vi "Begin.vi"() -> (1 "CameraDevRef":T5)   [LabVIEW 2011]
doc: "Called before other user functions, this VI is expected to open initial I/O refnums, load in file data, and do all program initialization. Notice that the <B>error out</B> terminal is simply used for data flow. Wiring it to other structures or subVIs ensures that this VI runs first."
uses:
  <vilib>/Rock Robotics/WPI/Camera/WPI_CameraDevRef.ctl
  <vilib>/Rock Robotics/WPI/Encoder/WPI_EncoderDevRef.ctl
  <vilib>/Rock Robotics/SystemInterfaces/Encoder/FPGA_EncoderIdx.ctl
  <vilib>/Rock Robotics/SystemInterfaces/Counter/FPGA_CounterCtrSystemIndex.ctl
  <vilib>/Rock Robotics/WPI/Encoder/WPI_EncoderType.ctl
  <vilib>/Rock Robotics/WPI/Joystick/WPI_JoystickDeviceEnum.ctl
  <vilib>/Rock Robotics/SystemInterfaces/DIO/FPGA_DIOPWMChannel.ctl
  <vilib>/Rock Robotics/SystemInterfaces/Typedef/FPGA_TypedefDigitalModule.ctl
  <vilib>/Rock Robotics/WPI/MotorControl/WPI_MotorControlOpen Victor.vi
  Robot Global Data.vi
  <vilib>/Rock Robotics/SystemInterfaces/DIO/FPGA_DIORelayChannel.ctl
  <vilib>/Rock Robotics/WPI/Relay/WPI_RelayDirection.ctl
  <vilib>/Rock Robotics/SystemInterfaces/AI/FPGA_AIChannel.ctl
  <vilib>/Rock Robotics/WPI/Counter/WPI_CounterDigitalInputToDigitalSource.vi
  <vilib>/Rock Robotics/SystemInterfaces/DIO/FPGA_DIOChannel.ctl
  <vilib>/Rock Robotics/SystemInterfaces/AI/FPGA_AIGyroChannel.ctl
  <vilib>/Rock Robotics/WPI/MotorControl/WPI_MotorControlOpen Jaguar.vi
  <vilib>/Rock Robotics/SystemInterfaces/Typedef/FPGA_TypedefAnalogModule.ctl
  <vilib>/Utility/file.llb/Read From Spreadsheet File (DBL).vi
panel:
  out "LDriveEncoder 3":cluster{"status":bool}
  out "EncoderDevRef 3":T1={"DevStatus"={"status"=FALSE, "code"=0, "source"=""}, "EncoderIndex"=enum."Invalid", "CounterIndex"=enum."Invalid", "DistancePerCount"=1.0, "Decoding Type"=enum."4x"}
  out "EncoderDevRef 2":T1={"DevStatus"={"status"=FALSE, "code"=0, "source"=""}, "EncoderIndex"=enum."Invalid", "CounterIndex"=enum."Invalid", "DistancePerCount"=1.0, "Decoding Type"=enum."4x"}
  out "LDriveEncoder 2":errorcluster
  out "EncoderDevRef":T1={"DevStatus"={"status"=FALSE, "code"=0, "source"=""}, "EncoderIndex"=enum."Invalid", "CounterIndex"=enum."Invalid", "DistancePerCount"=1.0, "Decoding Type"=enum."4x"}
  out "LDriveEncoder":errorcluster
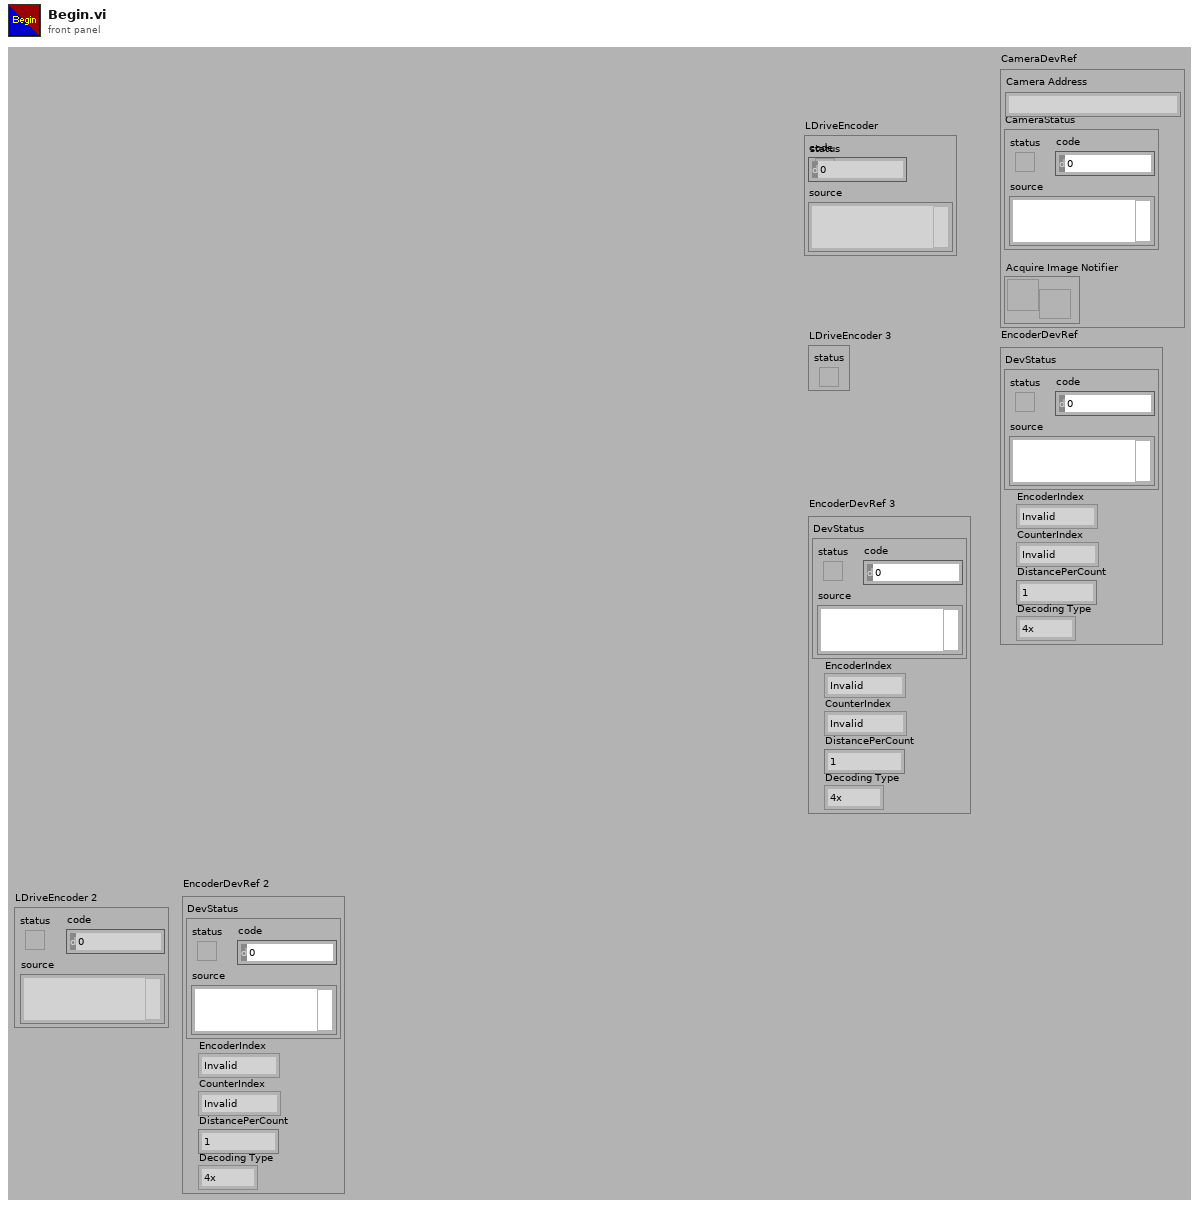
[diagram p1: front panel]
types:
  T1 = typedef "WPI_EncoderDevRef.ctl" = cluster{"DevStatus":errorcluster, "EncoderIndex":T2, "CounterIndex":T3, "DistancePerCount":dbl, "Decoding Type":T4}
  T2 = typedef "FPGA_EncoderIdx.ctl" = enum8{"Enc 0", "Enc 1", "Enc 2", "Enc 3", "Invalid"}
  T3 = typedef "FPGA_CounterCtrSystemIndex.ctl" = enum8{"Ctr 0", "Ctr 1", "Ctr 2", "Ctr 3", "Ctr 4", "Ctr 5", "Ctr 6", "Ctr 7", "Invalid"}
  T4 = typedef "WPI_EncoderType.ctl" = enum16{"1x", "2x", "4x"}
  T5 = typedef "WPI_CameraDevRef.ctl" = cluster{"Camera Address":string, "CameraStatus":errorcluster, "Acquire Image Notifier":refnum<notifier>}
  T6 = typedef "FPGA_TypedefDigitalModule.ctl" = enum16{"Digital Module 1", "Digital Module 2"}
  T7 = typedef "FPGA_DIOPWMChannel.ctl" = enum8{"PWM 1", "PWM 2", "PWM 3", "PWM 4", "PWM 5", "PWM 6", "PWM 7", "PWM 8", "PWM 9", "PWM 10", "Invalid"}
  T8 = typedef "WPI_JoystickDeviceEnum.ctl" = enum16{"USB 1", "USB 2", "USB 3", "USB 4", "Kinect 1", "Kinect 2"}
  T9 = typedef "FPGA_DIORelayChannel.ctl" = enum8{"Relay 1", "Relay 2", "Relay 3", "Relay 4", "Relay 5", "Relay 6", "Relay 7", "Relay 8", "Invalid"}
  T10 = typedef "FPGA_DIOChannel.ctl" = enum8{"DIO 1", "DIO 2", "DIO 3", "DIO 4", "DIO 5", "DIO 6", "DIO 7", "DIO 8", "DIO 9", "DIO 10", "DIO 11", "DIO 12", "DIO 13", "DIO 14", "Invalid"}
  T11 = typedef "WPI_MotorControlDeviceRef.ctl" = cluster{"DeviceStatus":errorcluster, "Type":enum16{"PWM", "CAN"}, "PWM":cluster{"Digital Module":T6, "PWM Channel":T7, "DeadBand":T12}, "CAN":cluster{"Device Number":u8, "Control Mode":T13, "Semaphore":T14, "Max Vout":dbl}, "Invert":bool, "TransformRef":T15, "InvTransformRef":T15}
  T12 = typedef "WPI_PWMDeadband.ctl" = cluster{"Name":string, "maxPositivePwm":i32, "minPositivePwm":i32, "centerPwm":i32, "maxNegativePwm":i32, "minNegativePwm":i32, "angularRange":u16}
  T13 = typedef "WPI_CANJaguar_ControlMode.ctl" = enum8{"Percent VBus", "Current", "Speed", "Position", "Voltage"}
  T14 = typedef "Semaphore RefNum" = refnum<k1>
  T15 = typedef "WPI_PWMTransform_ConPane.ctl" = refnum<vi>
  T16 = typedef "WPI_DigitalInputDevRef.ctl" = cluster{"DevStatus":errorcluster, "DIO Channel":T10, "Digital Module":T6}
  T17 = typedef "FPGA_CounterEncoderSourceConvertionLVSourceType.ctl" = cluster{"DevStatus":errorcluster, "AnalogTriggerMode?":bool, "DigitalMode":cluster{"Digital Module":T6, "DIO Channel":T18}, "AnalogTriggerMode":cluster{"AnalogTriggerIndex":T19, "OutputType":T20}}
  T18 = typedef "FPGA_DIODigitalSourceChannel.ctl" = enum8{"DIO 1", "DIO 2", "DIO 3", "DIO 4", "DIO 5", "DIO 6", "DIO 7", "DIO 8", "DIO 9", "DIO 10", "DIO 11", "DIO 12", "DIO 13", "DIO 14", "Disabled"}
  T19 = typedef "FPGA_AnalogTriggerIndex.ctl" = enum8{"Trig 0", "Trig 1", "Trig 2", "Trig 3", "Trig 4", "Trig 5", "Trig 6", "Trig 7", "Invalid"}
  T20 = typedef "FPGA_AnalogTriggerOutType.ctl" = enum16{"InWindow", "TriggerState", "Rising", "Falling"}
  T21 = typedef "WPI_RelayDevRef.ctl" = cluster{"DevStatus":errorcluster, "Relay Channel":T9, "Digital Module":T6, "Relay Direction":T22}
  T22 = typedef "WPI_RelayDirection.ctl" = enum16{"Both directions", "Forward only", "Reverse only"}
  T23 = typedef "FPGA_AIChannel.ctl" = enum8{"AI 1", "AI 2", "AI 3", "AI 4", "AI 5", "AI 6", "AI 7", "AI 8", "Invalid"}
  T24 = typedef "WPI_AnalogChannelDevRef.ctl" = cluster{"DevStatus":errorcluster, "Analog Module":T25, "Analog Channel":T23}
  T25 = typedef "FPGA_TypedefAnalogModule.ctl" = enum16{"Analog Module 1", "Analog Module 2"}
  T26 = typedef "WPI_CameraImageSize.ctl" = enum16{"640x480", "320x240", "160x120"}
  T27 = cluster{"fps":i32, "compression":i32, "Image Size":T26}
  T28 = typedef "WPI_CameraWhite Balance Values.ctl" = enum16{"Auto", "Fixed indoor", "Fixed outdoor 1", "Fixed outdoor 2", "Fixed fluorescent 1", "Fixed fluorescent 2", "Hold current"}
  T29 = typedef "WPI_CameraExposure Values.ctl" = enum16{"Auto", "Flicker-free 50 Hz", "Flicker-free 60 Hz", "Hold current"}
  T30 = typedef "WPI_ServoDeviceRef.ctl" = cluster{"DeviceStatus":errorcluster, "Digital Module":T6, "PWM Channel":T7, "DeadBand":T12}
  T31 = typedef "WPI_JoystickDevRef.ctl" = cluster{"Device":T8}
  T32 = typedef "FPGA_AIGyroChannel.ctl" = enum8{"AI 1", "AI 2", "Invalid"}
  T33 = typedef "WPI_GyroDevRef.ctl" = cluster{"DevStatus":errorcluster, "Analog Module":T25, "Analog Channel":T23, "Offset":dbl, "Gain (VoltsPerDegree/Second)":dbl}
  T34 = typedef "WPI_UltrasonicDeviceRef.ctl" = cluster{"DevStatus":errorcluster, "Ping Digital Module":T6, "Echo Digital Module":T6, "Ping Channel":T10, "Echo Channel":T10, "CntIndex":T3}
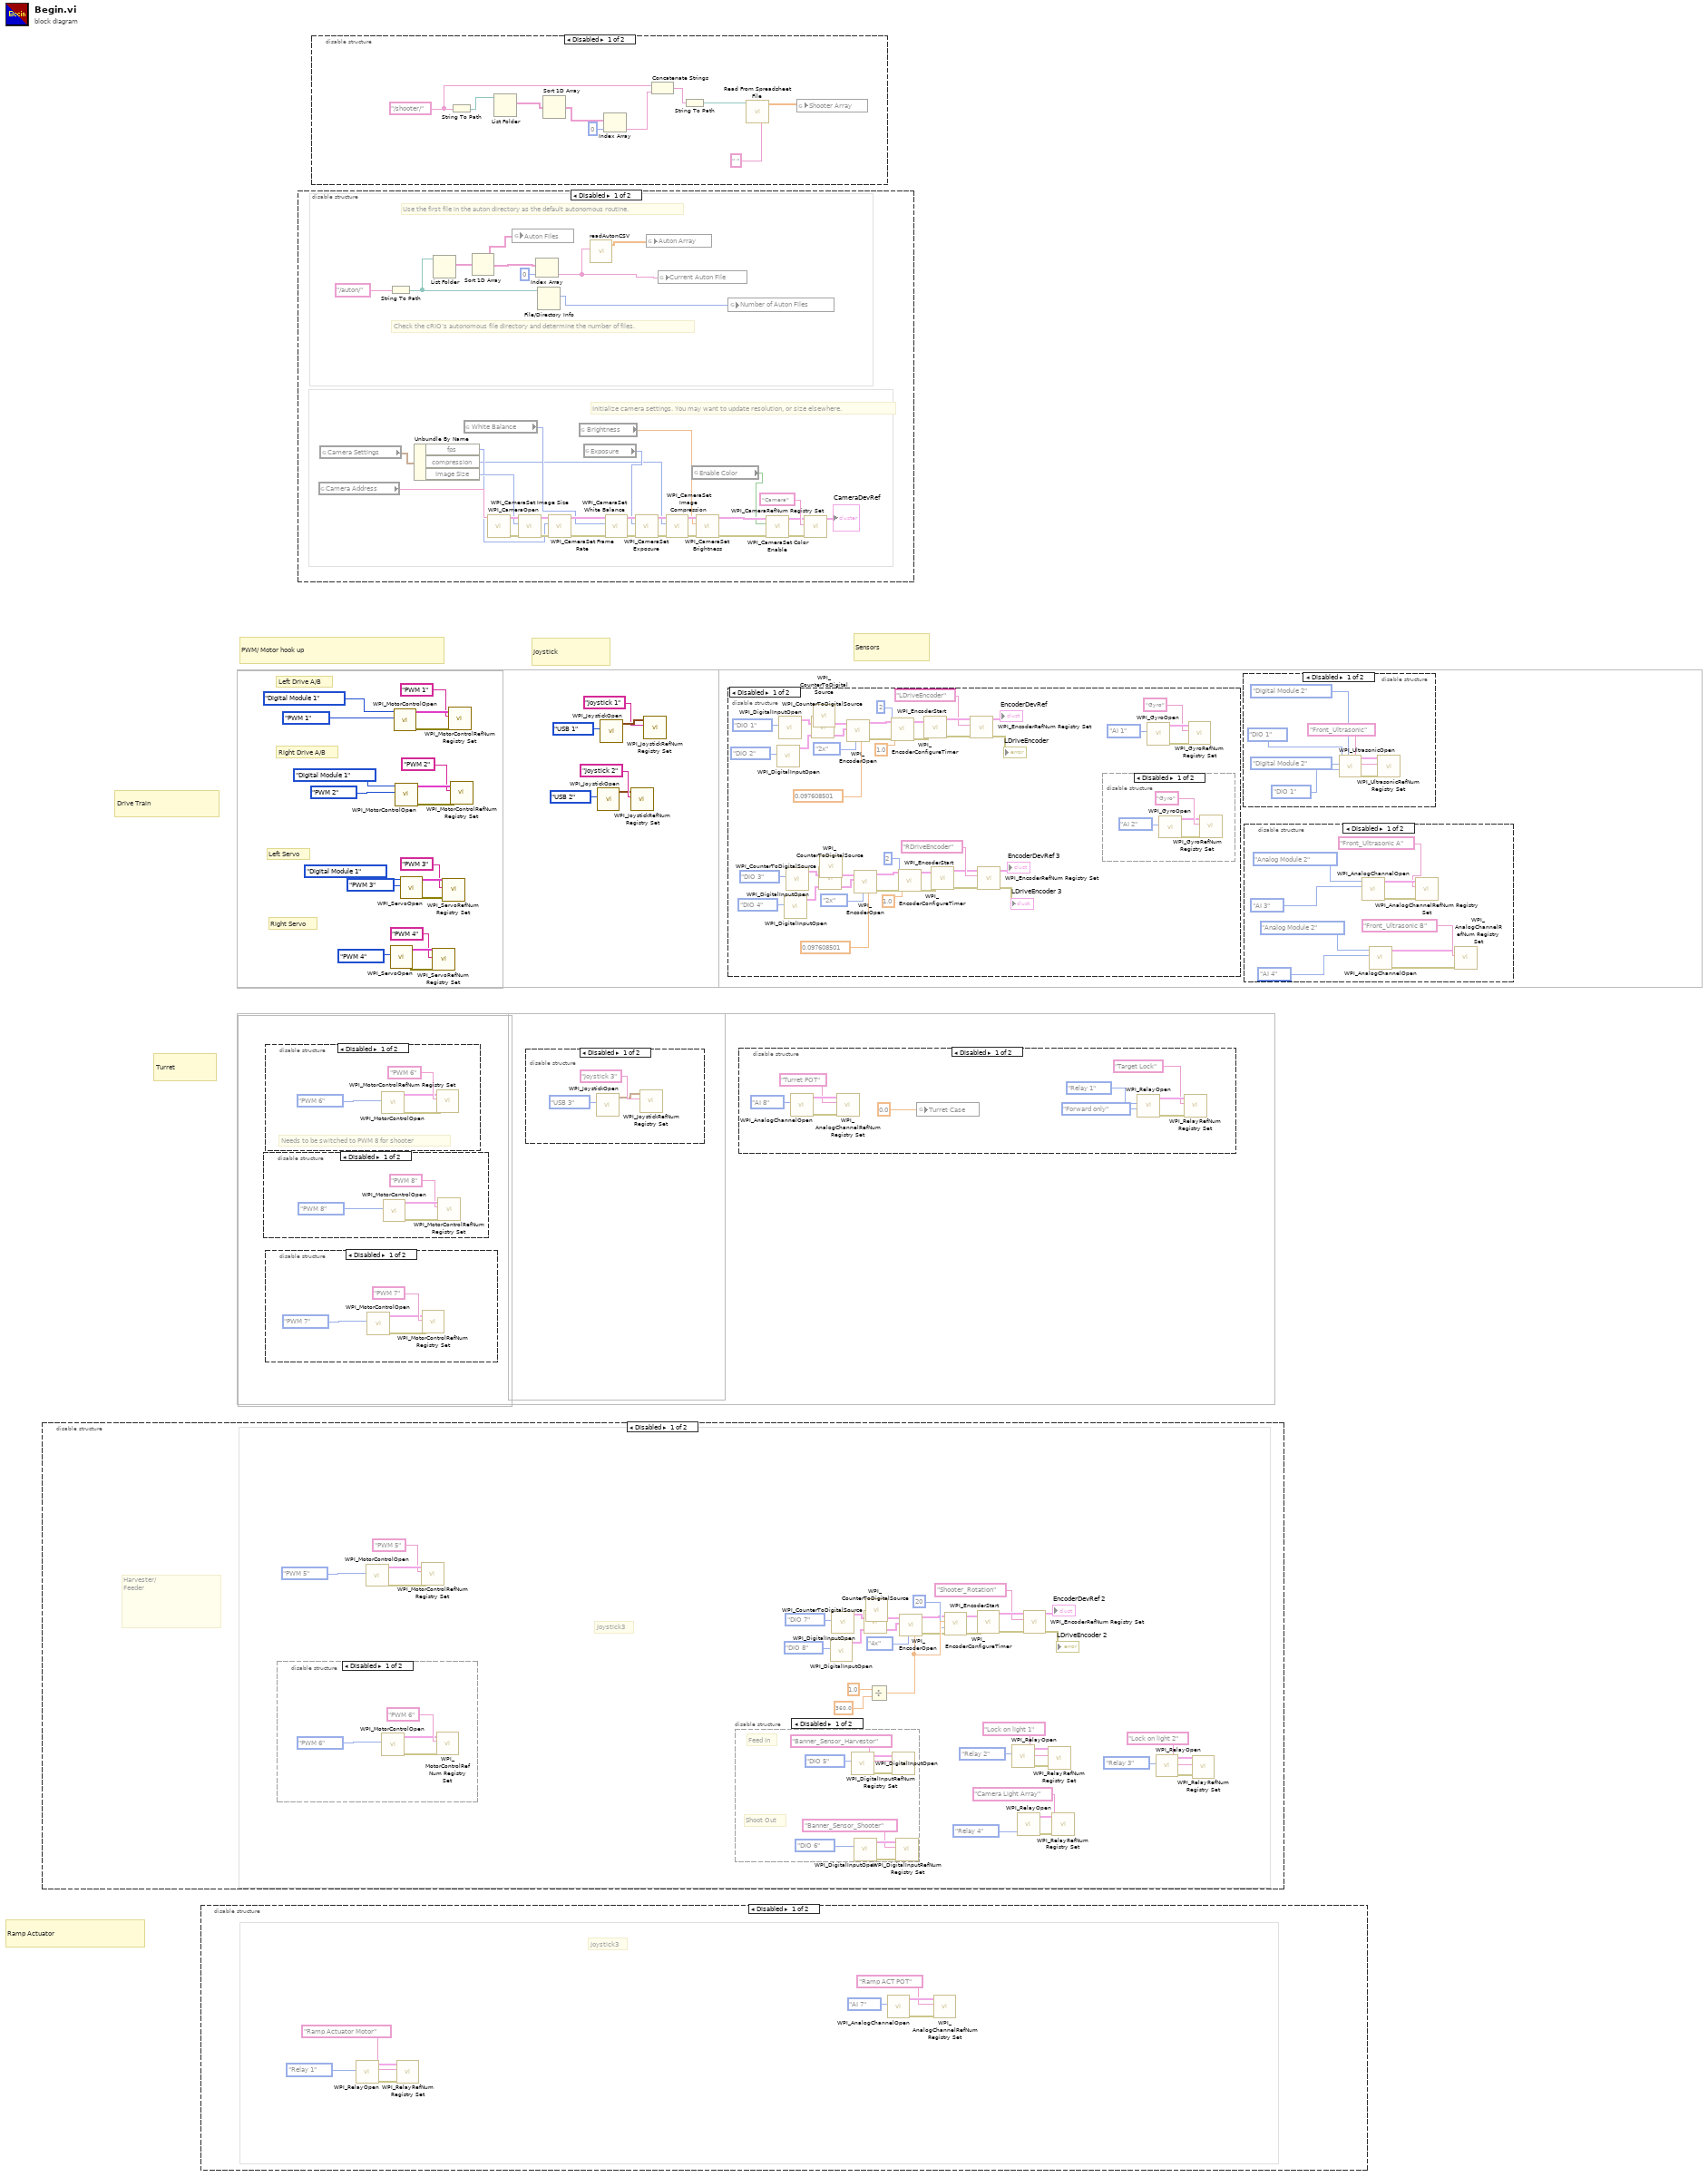
[diagram p0: block diagram]
diagram:
  # "Right Drive A/B"
  # "Left Drive A/B"
  # "Right Servo"
  # "Left Servo"
  # "Turret"
  # "Ramp Actuator"
  # "Drive Train"
  # "Sensors"
  # "Joystick"
  # "PWM/ Motor hook up"
  n1 = disable-structure shown="Disabled" {
    frame Disabled {
      # "Harvester/\nFeeder"
      # "Joystick3"
      n2 = disable-structure shown="Disabled" {
        frame Disabled {
          n3 = call-poly <vilib>:"WPI_MotorControlOpen.vi"("PWM Channel"=FPGA_DIOPWMChannel."PWM 6") -> ("error out"=w73:errorcluster, "MotorControlDeviceRef"=w71:T11)  [unwired: 9 in]
          n4 = call <vilib>:"WPI_MotorControlRefNum Registry Set.vi"("error in (no error)"=w73, "refnum name"="PWM 6", "MotorControlDevRef"=w71) -> ()  [unwired: 7 in, 2 out]
        }
        frame Enabled {
        }
      }
      n5 = call-poly <vilib>:"WPI_MotorControlOpen.vi"("PWM Channel"=FPGA_DIOPWMChannel."PWM 5") -> ("error out"=w58:errorcluster, "MotorControlDeviceRef"=w60:T11)  [unwired: 9 in]
      n6 = call <vilib>:"WPI_MotorControlRefNum Registry Set.vi"("error in (no error)"=w58, "refnum name"="PWM 5", "MotorControlDevRef"=w60) -> ()  [unwired: 7 in, 2 out]
      n7 = disable-structure shown="Disabled" {
        frame Disabled {
          # "Shoot Out"
          # "Feed in"
          n8 = call <vilib>:"WPI_DigitalInputOpen.vi"("DIO Channel"=FPGA_DIOChannel."DIO 5") -> ("error out"=w67:errorcluster, "DigitalInputDevRef"=w66:T16)  [unwired: 9 in]
          n9 = call <vilib>:"WPI_DigitalInputOpen.vi"("DIO Channel"=FPGA_DIOChannel."DIO 6") -> ("error out"=w64:errorcluster, "DigitalInputDevRef"=w63:T16)  [unwired: 9 in]
          n10 = call <vilib>:"WPI_DigitalInputRefNum Registry Set.vi"("error in (no error)"=w67, "refnum name"="Banner_Sensor_Harvestor", "DigitalInputDevRef"=w66) -> ()  [unwired: 7 in, 2 out]
          n11 = call <vilib>:"WPI_DigitalInputRefNum Registry Set.vi"("error in (no error)"=w64, "refnum name"="Banner_Sensor_Shooter", "DigitalInputDevRef"=w63) -> ()  [unwired: 7 in, 2 out]
        }
        frame Enabled {
        }
      }
      n12 = call <vilib>:"WPI_DigitalInputOpen.vi"("DIO Channel"=FPGA_DIOChannel."DIO 8") -> ("DigitalInputDevRef"=w42:T16)  [unwired: 9 in, 1 out]
      n13 = call <vilib>:"WPI_DigitalInputOpen.vi"("DIO Channel"=FPGA_DIOChannel."DIO 7") -> ("DigitalInputDevRef"=w39:T16)  [unwired: 9 in, 1 out]
      n14 = call-poly <vilib>:"WPI_CounterToDigitalSource.vi"("DigitalInputDevRef"=w42) -> ("Digital Source"=w43:T17)  [unwired: 6 in]
      n15 = call-poly <vilib>:"WPI_CounterToDigitalSource.vi"("DigitalInputDevRef"=w39) -> ("Digital Source"=w38:T17)  [unwired: 6 in]
      n16 = Divide(x=1.0, y=360.0) -> (x/y=w57:dbl)
      n17 = call <vilib>:"WPI_EncoderOpen.vi"("DistancePerCount"=w57, "Decoding Type"=WPI_EncoderType."4x", "BSource"=w43, "ASource"=w38) -> ("error out"=w46:errorcluster, "EncoderDevRef"=w47:T1)  [unwired: 6 in]
      n18 = call <vilib>:"WPI_EncoderConfigureTimer.vi"("error in (no error)"=w46, "Number Samples to Average"=u8 20, "Minimum Rate"=w57, "EncoderDevRef"=w47) -> ("error out"=w50:errorcluster, "EncoderDevRef"=w49:T1)  [unwired: 6 in]
      n19 = call <vilib>:"WPI_EncoderStart.vi"("error in (no error)"=w50, "EncoderDevRef"=w49) -> ("error out"=w52:errorcluster, "EncoderDevRef"=w51:T1)  [unwired: 8 in]
      n20 = call <vilib>:"WPI_RelayOpen.vi"("Relay Channel"=FPGA_DIORelayChannel."Relay 2") -> ("error out"=w35:errorcluster, "RelayDevRef"=w34:T21)  [unwired: 9 in]
      n21 = call <vilib>:"WPI_RelayOpen.vi"("Relay Channel"=FPGA_DIORelayChannel."Relay 4") -> ("error out"=w37:errorcluster, "RelayDevRef"=w36:T21)  [unwired: 9 in]
      n22 = call <vilib>:"WPI_EncoderRefNum Registry Set.vi"("error in (no error)"=w52, "refnum name"="Shooter_Rotation", "EncoderDevRef"=w51) -> ("error out"=→"LDriveEncoder 2":errorcluster, "EncoderDevRef"=→"EncoderDevRef 2":T1)  [unwired: 7 in]
      n23 = call <vilib>:"WPI_RelayRefNum Registry Set.vi"("error in (no error)"=w35, "refnum name"="Lock on light 1", "RelayDevRef"=w34) -> ()  [unwired: 7 in, 2 out]
      n24 = call <vilib>:"WPI_RelayRefNum Registry Set.vi"("error in (no error)"=w37, "refnum name"="Camera Light Array", "RelayDevRef"=w36) -> ()  [unwired: 7 in, 2 out]
      n25 = call <vilib>:"WPI_RelayOpen.vi"("Relay Channel"=FPGA_DIORelayChannel."Relay 3") -> ("error out"=w26:errorcluster, "RelayDevRef"=w27:T21)  [unwired: 9 in]
      n26 = call <vilib>:"WPI_RelayRefNum Registry Set.vi"("error in (no error)"=w26, "refnum name"="Lock on light 2", "RelayDevRef"=w27) -> ()  [unwired: 7 in, 2 out]
    }
    frame Enabled {
    }
  }
  n27 = disable-structure shown="Disabled" {
    frame Disabled {
      # "Joystick3"
      n28 = call <vilib>:"WPI_RelayOpen.vi"("Relay Channel"=FPGA_DIORelayChannel."Relay 1") -> ("error out"=w77:errorcluster, "RelayDevRef"=w76:T21)  [unwired: 9 in]
      n29 = call <vilib>:"WPI_RelayRefNum Registry Set.vi"("error in (no error)"=w77, "refnum name"="Ramp Actuator Motor", "RelayDevRef"=w76) -> ()  [unwired: 7 in, 2 out]
      n30 = call <vilib>:"WPI_AnalogChannelOpen.vi"("Analog Channel"=FPGA_AIChannel."AI 7") -> ("error out"=w80:errorcluster, "AIDeviceRef"=w81:T24)  [unwired: 9 in]
      n31 = call <vilib>:"WPI_AnalogChannelRefNum Registry Set.vi"("error in (no error)"=w80, "refnum name"="Ramp ACT POT", "AIDeviceRef"=w81) -> ()  [unwired: 7 in, 2 out]
    }
    frame Enabled {
    }
  }
  n32 = disable-structure shown="Disabled" {
    frame Disabled {
      n33 = call-poly <vilib>:"WPI_MotorControlOpen.vi"("PWM Channel"=FPGA_DIOPWMChannel."PWM 8") -> ("error out"=w82:errorcluster, "MotorControlDeviceRef"=w84:T11)  [unwired: 9 in]
      n34 = call <vilib>:"WPI_MotorControlRefNum Registry Set.vi"("error in (no error)"=w82, "refnum name"="PWM 8", "MotorControlDevRef"=w84) -> ()  [unwired: 7 in, 2 out]
    }
    frame Enabled {
    }
  }
  n35 = disable-structure shown="Disabled" {
    frame Disabled {
      # "Needs to be switched to PWM 8 for shooter"
      n36 = call-poly <vilib>:"WPI_MotorControlOpen.vi"("PWM Channel"=FPGA_DIOPWMChannel."PWM 6") -> ("error out"=w89:errorcluster, "MotorControlDeviceRef"=w87:T11)  [unwired: 9 in]
      n37 = call <vilib>:"WPI_MotorControlRefNum Registry Set.vi"("error in (no error)"=w89, "refnum name"="PWM 6", "MotorControlDevRef"=w87) -> ()  [unwired: 7 in, 2 out]
    }
    frame Enabled {
    }
  }
  n38 = disable-structure shown="Disabled" {
    frame Disabled {
      n39 = call-poly <vilib>:"WPI_MotorControlOpen.vi"("PWM Channel"=FPGA_DIOPWMChannel."PWM 7") -> ("error out"=w93:errorcluster, "MotorControlDeviceRef"=w91:T11)  [unwired: 9 in]
      n40 = call <vilib>:"WPI_MotorControlRefNum Registry Set.vi"("error in (no error)"=w93, "refnum name"="PWM 7", "MotorControlDevRef"=w91) -> ()  [unwired: 7 in, 2 out]
    }
    frame Enabled {
    }
  }
  n41 = disable-structure shown="Disabled" {
    frame Disabled {
      # "Check the cRIO's autonomous file directory and determine the number of files."
      # "Use the first file in the auton directory as the default autonomous routine."
      # "Initialize camera settings. You may want to update resolution, or size elsewhere."
      n42 = global read "Robot Global Data.vi" "Camera Address"() -> (w115:string)
      n43 = global read "Robot Global Data.vi" "Camera Settings"() -> (w114:T27)
      n44 = String To Path(string="/auton/") -> (path=w100:path)
      n45 = Unbundle By Name(w114) -> ("fps"=w112:i32, "compression"=w109:i32, "Image Size"=w113:T26)
      n46 = List Folder(path=w100) -> (filenames=w99:string[])  [unwired: 1 in, 5 out]
      n47 = global read "Robot Global Data.vi" "White Balance"() -> (w111:T28)
      n48 = Sort 1D Array(array=w99) -> (sorted array=w94:string[])
      n49 = call <vilib>:"WPI_CameraOpen.vi"("Camera Address"=w115) -> ("error out"=w121:errorcluster, "CameraDevRef"=w122:T5)  [unwired: 1 in, 8 out]
      n50 = global write "Robot Global Data.vi" "Auton Files"(w94) -> ()
      n51 = call <vilib>:"WPI_CameraSet Image Size.vi"("error in (no error)"=w121, "Image Size"=w113, "CameraDevRef"=w122) -> ("error out"=w120:errorcluster, "CameraDevRef Out"=w123:T5)  [unwired: 7 out]
      n52 = Index Array(array=w94, index=0) -> (element=w96:string)
      n53 = File/Directory Info(path=w100) -> (size=w97:i64)  [unwired: 1 in, 6 out]
      n54 = call <vilib>:"WPI_CameraSet Frame Rate.vi"("error in (no error)"=w120, "Frame Rate (fps)"=w112, "CameraDevRef"=w123) -> ("error out"=w119:errorcluster, "CameraDevRef Out"=w125:T5)  [unwired: 7 out]
      n55 = global read "Robot Global Data.vi" "Brightness"() -> (w108:dbl)
      n56 = global read "Robot Global Data.vi" "Exposure"() -> (w110:T29)
      n57 = call "readAutonCSV.vi"("AutonFile"=w96) -> ("AutonArray"=w95:dbl[][])  [unwired: 7 in]
      n58 = call <vilib>:"WPI_CameraSet White Balance.vi"("error in (no error)"=w119, "White Balance"=w111, "CameraDevRef"=w125) -> ("error out"=w118:errorcluster, "CameraDevRef Out"=w124:T5)  [unwired: 7 out]
      n59 = call <vilib>:"WPI_CameraSet Exposure.vi"("error in (no error)"=w118, "Exposure"=w110, "CameraDevRef"=w124) -> ("error out"=w117:errorcluster, "CameraDevRef Out"=w127:T5)  [unwired: 7 out]
      n60 = global write "Robot Global Data.vi" "Auton Array"(w95) -> ()
      n61 = global write "Robot Global Data.vi" "Current Auton File"(w96) -> ()
      n62 = call <vilib>:"WPI_CameraSet Image Compression.vi"("error in (no error)"=w117, "Compression"=w109, "CameraDevRef"=w127) -> ("error out"=w116:errorcluster, "CameraDevRef Out"=w126:T5)  [unwired: 7 out]
      n63 = global read "Robot Global Data.vi" "Enable Color"() -> (w103:bool)
      n64 = call <vilib>:"WPI_CameraSet Brightness.vi"("error in (no error)"=w116, "Brightness"=w108, "CameraDevRef"=w126) -> ("error out"=w106:errorcluster, "CameraDevRef Out"=w107:T5)  [unwired: 7 out]
      n65 = global write "Robot Global Data.vi" "Number of Auton Files"(w97) -> ()
      n66 = call <vilib>:"WPI_CameraSet Color Enable.vi"("error in (no error)"=w106, "Color Enabled"=w103, "CameraDevRef"=w107) -> ("error out"=w104:errorcluster, "CameraDevRef Out"=w105:T5)  [unwired: 7 in]
      n67 = call <vilib>:"WPI_CameraRefNum Registry Set.vi"("error in (no error)"=w104, "refnum name"="Camera", "CameraDevRef"=w105) -> ("CameraDevRef"=→"CameraDevRef":T5)  [unwired: 8 out]
    }
    frame Enabled {
    }
  }
  n68 = disable-structure shown="Disabled" {
    frame Disabled {
      w137 = "/shooter/" ("string")
      n69 = String To Path(string=w137) -> (path=w138:path)
      n70 = List Folder(path=w138) -> (filenames=w136:string[])  [unwired: 1 in, 5 out]
      n71 = Sort 1D Array(array=w136) -> (sorted array=w135:string[])
      n72 = Index Array(array=w135, index=0) -> (element=w133:string)
      n73 = Concatenate Strings(w137, w133) -> (w132:string)
      n74 = String To Path(string=w132) -> (path=w131:path)
      n75 = call-poly <vilib>:"Read From Spreadsheet File.vi"("delimiter (\\t)"=" " ("delimiter (\\t)"), "file path (dialog if empty)"=w131) -> ("all rows"=w129:dbl[][])  [unwired: 5 in, 4 out]
      n76 = global write "Robot Global Data.vi" "Shooter Array"(w129) -> ()
    }
    frame Enabled {
    }
  }
  n77 = call <vilib>:"WPI_ServoOpen.vi"("PWM Channel"=FPGA_DIOPWMChannel."PWM 4") -> ("error out"=w1:errorcluster, "ServoDeviceRef"=w16:T30)  [unwired: 9 in]
  n78 = call-poly <vilib>:"WPI_MotorControlOpen.vi"("PWM Channel"=FPGA_DIOPWMChannel."PWM 1", "Digital Module (Module 1)"=FPGA_TypedefDigitalModule."Digital Module 1") -> ("error out"=w6:errorcluster, "MotorControlDeviceRef"=w9:T11)  [unwired: 8 in]
  n79 = call-poly <vilib>:"WPI_MotorControlOpen.vi"("PWM Channel"=FPGA_DIOPWMChannel."PWM 2", "Digital Module (Module 1)"=FPGA_TypedefDigitalModule."Digital Module 1") -> ("error out"=w7:errorcluster, "MotorControlDeviceRef"=w12:T11)  [unwired: 8 in]
  n80 = call <vilib>:"WPI_ServoOpen.vi"("PWM Channel"=FPGA_DIOPWMChannel."PWM 3", "Digital Module (Module 1)"=FPGA_TypedefDigitalModule."Digital Module 1") -> ("error out"=w2:errorcluster, "ServoDeviceRef"=w18:T30)  [unwired: 8 in]
  n81 = call <vilib>:"WPI_ServoRefNum Registry Set.vi"("error in (no error)"=w1, "refnum name"="PWM 4", "ServoDeviceRef"=w16) -> ()  [unwired: 7 in, 2 out]
  n82 = call <vilib>:"WPI_ServoRefNum Registry Set.vi"("error in (no error)"=w2, "refnum name"="PWM 3", "ServoDeviceRef"=w18) -> ()  [unwired: 7 in, 2 out]
  n83 = call <vilib>:"WPI_MotorControlRefNum Registry Set.vi"("error in (no error)"=w6, "refnum name"="PWM 1", "MotorControlDevRef"=w9) -> ()  [unwired: 7 in, 2 out]
  n84 = call <vilib>:"WPI_MotorControlRefNum Registry Set.vi"("error in (no error)"=w7, "refnum name"="PWM 2", "MotorControlDevRef"=w12) -> ()  [unwired: 7 in, 2 out]
  n85 = disable-structure shown="Disabled" {
    frame Disabled {
      n86 = call <vilib>:"WPI_JoystickOpen.vi"("JoystickDevice"=WPI_JoystickDeviceEnum."USB 3") -> ("JoystickDevRef"=w140:T31)  [unwired: 10 in]
      n87 = call <vilib>:"WPI_JoystickRefNum Registry Set.vi"("refnum name"="Joystick 3", "JoystickDevRef"=w140) -> ()  [unwired: 8 in, 2 out]
    }
    frame Enabled {
    }
  }
  n88 = call <vilib>:"WPI_JoystickOpen.vi"("JoystickDevice"=WPI_JoystickDeviceEnum."USB 2") -> ("JoystickDevRef"=w22:T31)  [unwired: 10 in]
  n89 = call <vilib>:"WPI_JoystickOpen.vi"("JoystickDevice"=WPI_JoystickDeviceEnum."USB 1") -> ("JoystickDevRef"=w25:T31)  [unwired: 10 in]
  n90 = call <vilib>:"WPI_JoystickRefNum Registry Set.vi"("refnum name"="Joystick 2", "JoystickDevRef"=w22) -> ()  [unwired: 8 in, 2 out]
  n91 = call <vilib>:"WPI_JoystickRefNum Registry Set.vi"("refnum name"="Joystick 1", "JoystickDevRef"=w25) -> ()  [unwired: 8 in, 2 out]
  n92 = disable-structure shown="Disabled" {
    frame Disabled {
      n93 = call <vilib>:"WPI_DigitalInputOpen.vi"("DIO Channel"=FPGA_DIOChannel."DIO 2") -> ("DigitalInputDevRef"=w165:T16)  [unwired: 9 in, 1 out]
      n94 = call <vilib>:"WPI_DigitalInputOpen.vi"("DIO Channel"=FPGA_DIOChannel."DIO 1") -> ("DigitalInputDevRef"=w162:T16)  [unwired: 9 in, 1 out]
      n95 = call <vilib>:"WPI_DigitalInputOpen.vi"("DIO Channel"=FPGA_DIOChannel."DIO 4") -> ("DigitalInputDevRef"=w156:T16)  [unwired: 9 in, 1 out]
      n96 = call <vilib>:"WPI_DigitalInputOpen.vi"("DIO Channel"=FPGA_DIOChannel."DIO 3") -> ("DigitalInputDevRef"=w159:T16)  [unwired: 9 in, 1 out]
      n97 = call-poly <vilib>:"WPI_CounterToDigitalSource.vi"("DigitalInputDevRef"=w165) -> ("Digital Source"=w166:T17)  [unwired: 6 in]
      n98 = call-poly <vilib>:"WPI_CounterToDigitalSource.vi"("DigitalInputDevRef"=w162) -> ("Digital Source"=w161:T17)  [unwired: 6 in]
      n99 = call-poly <vilib>:"WPI_CounterToDigitalSource.vi"("DigitalInputDevRef"=w156) -> ("Digital Source"=w155:T17)  [unwired: 6 in]
      n100 = call-poly <vilib>:"WPI_CounterToDigitalSource.vi"("DigitalInputDevRef"=w159) -> ("Digital Source"=w160:T17)  [unwired: 6 in]
      n101 = call <vilib>:"WPI_EncoderOpen.vi"("DistancePerCount"=0.097608501, "Decoding Type"=WPI_EncoderType."2x", "BSource"=w166, "ASource"=w161) -> ("error out"=w170:errorcluster, "EncoderDevRef"=w171:T1)  [unwired: 6 in]
      n102 = call <vilib>:"WPI_EncoderOpen.vi"("DistancePerCount"=0.097608501, "Decoding Type"=WPI_EncoderType."2x", "BSource"=w155, "ASource"=w160) -> ("error out"=w151:errorcluster, "EncoderDevRef"=w150:T1)  [unwired: 6 in]
      n103 = call <vilib>:"WPI_EncoderConfigureTimer.vi"("error in (no error)"=w170, "Number Samples to Average"=u8 2, "Minimum Rate"=1.0, "EncoderDevRef"=w171) -> ("error out"=w175:errorcluster, "EncoderDevRef"=w174:T1)  [unwired: 6 in]
      n104 = call <vilib>:"WPI_EncoderConfigureTimer.vi"("error in (no error)"=w151, "Number Samples to Average"=u8 2, "Minimum Rate"=1.0, "EncoderDevRef"=w150) -> ("error out"=w146:errorcluster, "EncoderDevRef"=w147:T1)  [unwired: 6 in]
      n105 = call <vilib>:"WPI_EncoderStart.vi"("error in (no error)"=w175, "EncoderDevRef"=w174) -> ("error out"=w177:errorcluster, "EncoderDevRef"=w176:T1)  [unwired: 8 in]
      n106 = call <vilib>:"WPI_EncoderStart.vi"("error in (no error)"=w146, "EncoderDevRef"=w147) -> ("error out"=w144:errorcluster, "EncoderDevRef"=w145:T1)  [unwired: 8 in]
      n107 = call <vilib>:"WPI_EncoderRefNum Registry Set.vi"("error in (no error)"=w177, "refnum name"="LDriveEncoder", "EncoderDevRef"=w176) -> ("error out"=→"LDriveEncoder":errorcluster, "EncoderDevRef"=→"EncoderDevRef":T1)  [unwired: 7 in]
      n108 = call <vilib>:"WPI_EncoderRefNum Registry Set.vi"("error in (no error)"=w144, "refnum name"="RDriveEncoder", "EncoderDevRef"=w145) -> ("error out"=→"LDriveEncoder 3":errorcluster, "EncoderDevRef"=→"EncoderDevRef 3":T1)  [unwired: 7 in]
      n109 = disable-structure shown="Disabled" {
        frame Disabled {
          n110 = call <vilib>:"WPI_GyroOpen.vi"("Analog Channel"=FPGA_AIGyroChannel."AI 2") -> ("error out"=w184:errorcluster, "GyroDevRef"=w185:T33)  [unwired: 8 in, 1 out]
          n111 = call <vilib>:"WPI_GyroRefNum Registry Set.vi"("error in (no error)"=w184, "refnum name"="Gyro", "GyroDevRef"=w185) -> ()  [unwired: 7 in, 2 out]
        }
        frame Enabled {
        }
      }
      n112 = call <vilib>:"WPI_GyroOpen.vi"("Analog Channel"=FPGA_AIGyroChannel."AI 1") -> ("error out"=w183:errorcluster, "GyroDevRef"=w182:T33)  [unwired: 8 in, 1 out]
      n113 = call <vilib>:"WPI_GyroRefNum Registry Set.vi"("error in (no error)"=w183, "refnum name"="Gyro", "GyroDevRef"=w182) -> ()  [unwired: 7 in, 2 out]
    }
    frame Enabled {
    }
  }
  n114 = disable-structure shown="Disabled" {
    frame Disabled {
      n115 = call <vilib>:"WPI_AnalogChannelOpen.vi"("Analog Channel"=FPGA_AIChannel."AI 8") -> ("error out"=w191:errorcluster, "AIDeviceRef"=w192:T24)  [unwired: 9 in]
      n116 = call <vilib>:"WPI_AnalogChannelRefNum Registry Set.vi"("error in (no error)"=w191, "refnum name"="Turret POT", "AIDeviceRef"=w192) -> ()  [unwired: 7 in, 2 out]
      n117 = global write "Robot Global Data.vi" "Turret Case"(0.0 ("Return To Home Case")) -> ()
      n118 = call <vilib>:"WPI_RelayOpen.vi"("Relay Direction"=WPI_RelayDirection."Forward only", "Relay Channel"=FPGA_DIORelayChannel."Relay 1") -> ("error out"=w196:errorcluster, "RelayDevRef"=w197:T21)  [unwired: 8 in]
      n119 = call <vilib>:"WPI_RelayRefNum Registry Set.vi"("error in (no error)"=w196, "refnum name"="Target Lock", "RelayDevRef"=w197) -> ()  [unwired: 7 in, 2 out]
    }
    frame Enabled {
    }
  }
  n120 = disable-structure shown="Disabled" {
    frame Disabled {
      n121 = call <vilib>:"WPI_UltrasonicOpen.vi"("Ping Digital Module (Module 1)"=FPGA_TypedefDigitalModule."Digital Module 2", "Echo DIO Channel"=FPGA_DIOChannel."DIO 1", "Echo Digital Module (Module 1)"=FPGA_TypedefDigitalModule."Digital Module 2", "Ping DIO Channel"=FPGA_DIOChannel."DIO 1") -> ("error out"=w204:errorcluster, "UltrasonicDevRef"=w203:T34)  [unwired: 6 in]
      n122 = call <vilib>:"WPI_UltrasonicRefNum Registry Set.vi"("error in (no error)"=w204, "refnum name"="Front_Ultrasonic", "UltrasonicDevRef"=w203) -> ()  [unwired: 7 in, 2 out]
    }
    frame Enabled {
    }
  }
  n123 = disable-structure shown="Disabled" {
    frame Disabled {
      n124 = call <vilib>:"WPI_AnalogChannelOpen.vi"("Analog Channel"=FPGA_AIChannel."AI 3", "Analog Module (Module 1)"=FPGA_TypedefAnalogModule."Analog Module 2") -> ("error out"=w210:errorcluster, "AIDeviceRef"=w209:T24)  [unwired: 8 in]
      n125 = call <vilib>:"WPI_AnalogChannelOpen.vi"("Analog Channel"=FPGA_AIChannel."AI 4", "Analog Module (Module 1)"=FPGA_TypedefAnalogModule."Analog Module 2") -> ("error out"=w205:errorcluster, "AIDeviceRef"=w206:T24)  [unwired: 8 in]
      n126 = call <vilib>:"WPI_AnalogChannelRefNum Registry Set.vi"("error in (no error)"=w210, "refnum name"="Front_Ultrasonic A", "AIDeviceRef"=w209) -> ()  [unwired: 7 in, 2 out]
      n127 = call <vilib>:"WPI_AnalogChannelRefNum Registry Set.vi"("error in (no error)"=w205, "refnum name"="Front_Ultrasonic B", "AIDeviceRef"=w206) -> ()  [unwired: 7 in, 2 out]
    }
    frame Enabled {
    }
  }
